vi "Pre Launch Init.vi"(11 "Sample in":refnum<class "Sample.lvclass">) -> (0 "error out":errorcluster, 3 "Sample out":refnum<class "Sample.lvclass">)   [LabVIEW 2022 SP3, in "Sample.lvlib" / "Sample.lvclass"]
doc: "(<B>Filename</B>: Actor Framework.lvlib:Actor.lvclass:Pre Launch Init.vi)\n\nDefines behavior that occurs after the Launch Actor method is invoked but before the actor's Actor Core method begins running.\n\nThe Pre Launch Init method is guaranteed to finish before the Launch Actor method returns to its caller and before the actor itself receives any messages. Any references that the Pre Launch Init method obtains are guaranteed to have the same lifetime as the actor itself. Any errors that the Pre Launch Init method returns will abort the launch.\n\nBy default, this method does nothing. A descendant class may override it to define behavior."
uses:
  Sample.lvclass
  Sample.lvclass/Sample.ctl
  <vilib>/MGI/Monitored Actor/Monitored Actor/Monitored Actor/Monitored Actor.lvclass
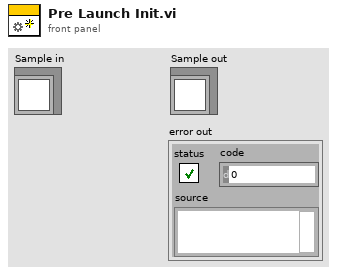
[diagram p1: front panel]
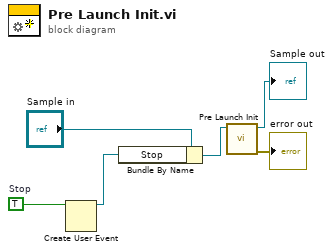
[diagram p0: block diagram]
diagram:
  w5 = TRUE  # Stop
  n1 = Create User Event(user event datatype=w5) -> (user event=w3:refnum<user-event>)  [unwired: 1 in, 1 out]
  n2 = Bundle By Name(cluster="Sample in", "Stop"=w3) -> (w2:refnum<class "Sample.lvclass">)
  n3 = call-parent "Pre Launch Init.vi"("Monitored Actor in"=w2) -> ("error out"=→"error out":errorcluster, "Monitored Actor out"=→"Sample out":refnum<class "Sample.lvclass">)  [unwired: 9 in]
